vi "Program12.vi"() -> ()   [LabVIEW 2020]
panel:
  in  "stop":bool
  out "Zdarzenia":string
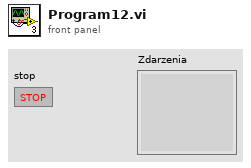
[diagram p1: front panel]
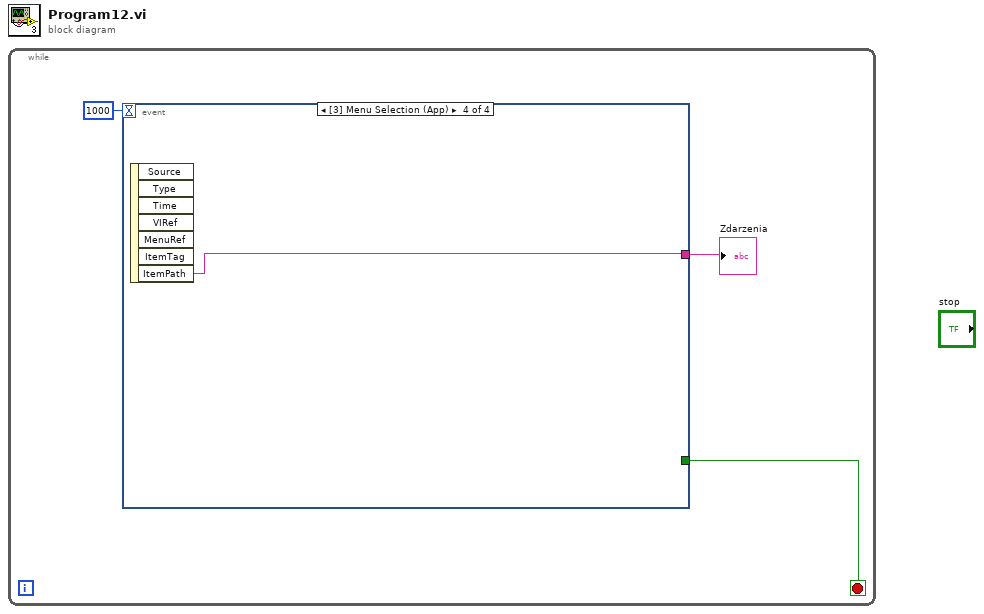
[diagram p0: block diagram]
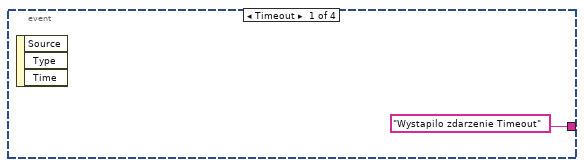
[diagram p2: hidden frame]
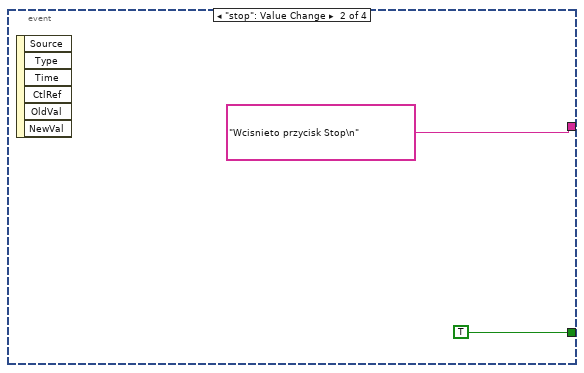
[diagram p3: hidden frame]
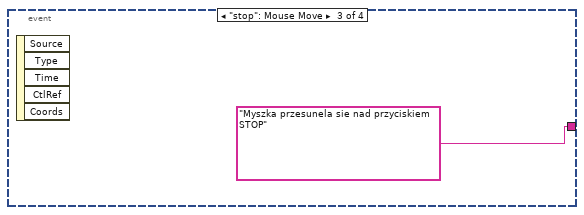
[diagram p4: hidden frame]
diagram:
  n1 = while {
    stop <- w1 stop-if-true
    n2 = event shown="[3] Menu Selection (App)" {
      selector: _ -> [_ _ _ _]
      dyn-events: _ -> [_ _ _ _]
      timeout: 1000 -> [_ _ _ _]
      tunnel: ["Wystapilo zdarzenie Timeout" "Wcisnieto przycisk Stop\n" "Myszka przesunela sie nad przyciskiem STOP" w8] -> w2
      tunnel: [_ TRUE _ _] -> w1
      event Timeout {
        n3 = event-data() -> ()  [unwired: 1 in, 3 out]
      }
      event "stop": Value Change {
        n4 = event-data() -> ()  [unwired: 1 in, 6 out]
      }
      event "stop": Mouse Move {
        n5 = event-data() -> ()  [unwired: 1 in, 5 out]
      }
      event Menu Selection (App) {
        n6 = event-data() -> ("ItemPath"=w8:string)  [unwired: 1 in, 6 out]
      }
    }
    "Zdarzenia" <- w2
  }
